vi "zad_14.vi"() -> ()   [LabVIEW 2024]
uses:
  Data_14.ctl
  <vilib>/regexp/Match Regular Expression.xnode
panel:
  out "error out":errorcluster
  in  "error in":errorcluster
  out "Limit exceeded?":bool
  out "To be moved":string
  in  "Sound intensity: MAX":dbl=100.0
  in  "Sound intensity: MIN":dbl
  in  "Stop":bool
  in  "Sound intensity [dB]":dbl(slide) scale=0.0..100.0
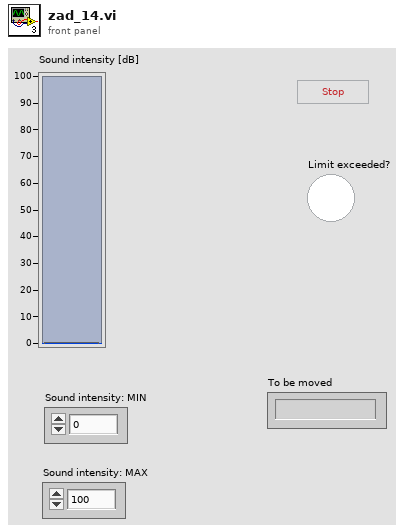
[diagram p1: front panel]
types:
  T1 = typedef "Data_14.ctl" = cluster{"Left":i32, "Top":i32, "Dragging":bool, "Letters":string}
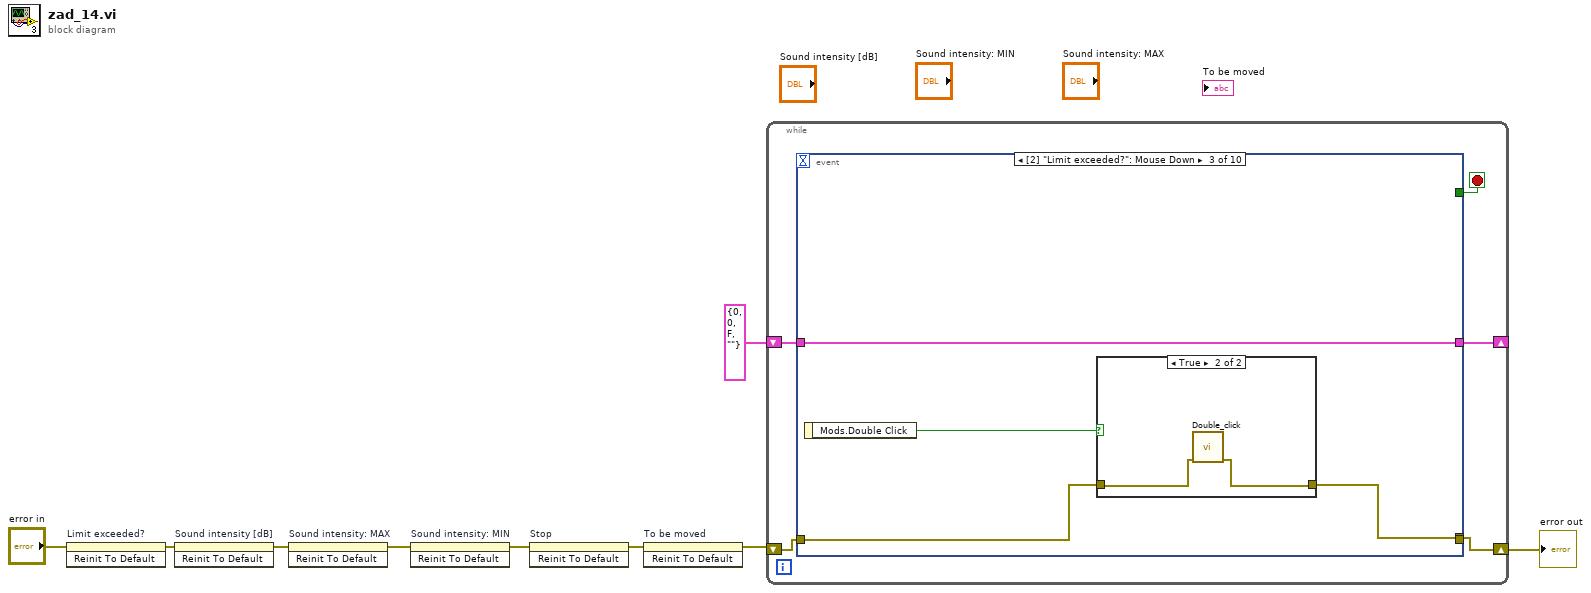
[diagram p0: block diagram]
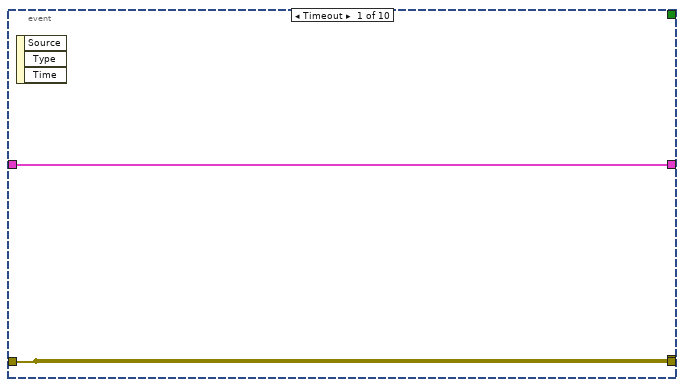
[diagram p2: hidden frame]
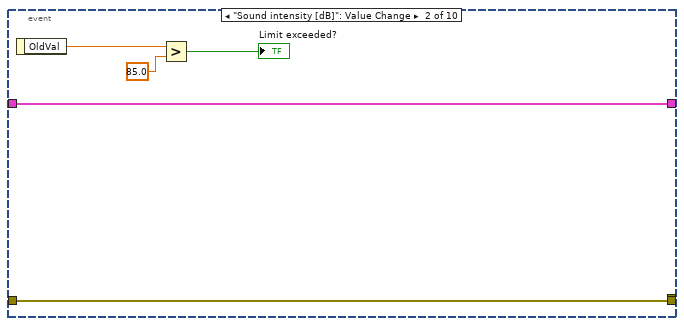
[diagram p3: hidden frame]
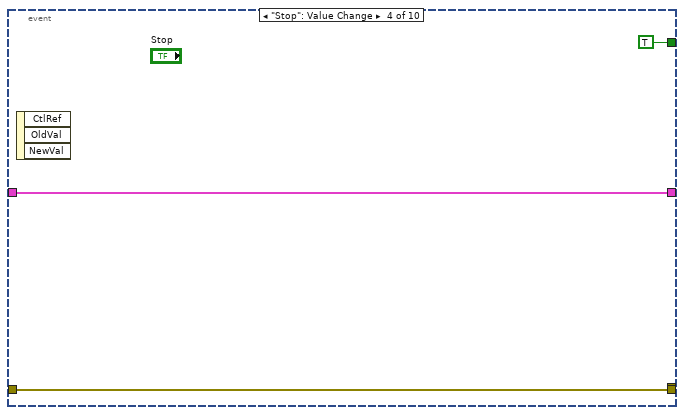
[diagram p5: hidden frame]
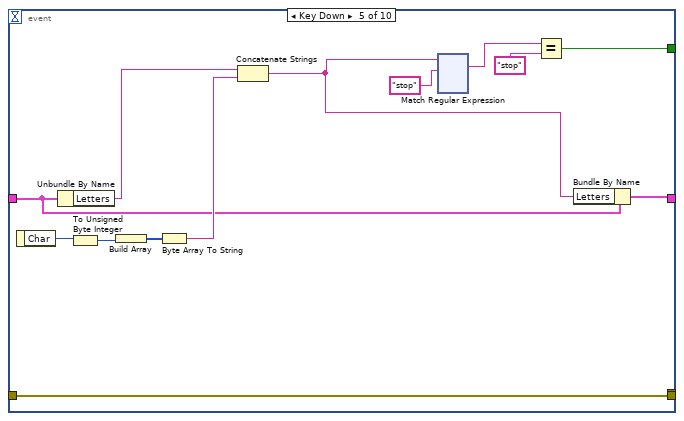
[diagram p6: hidden frame]
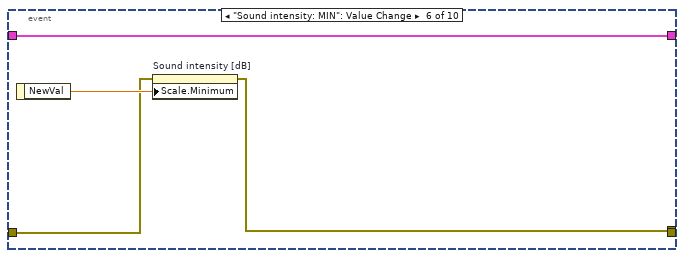
[diagram p7: hidden frame]
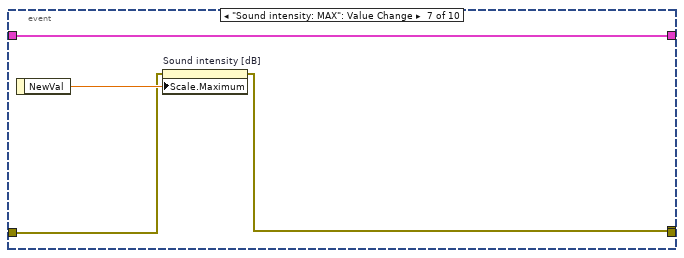
[diagram p8: hidden frame]
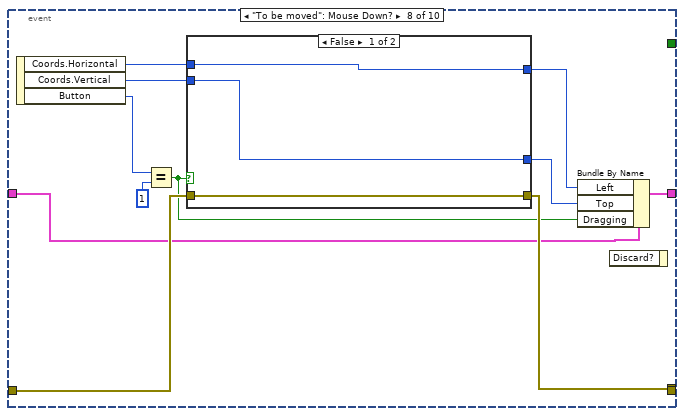
[diagram p9: hidden frame]
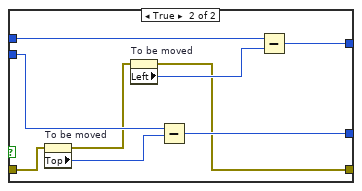
[diagram p10: hidden frame]
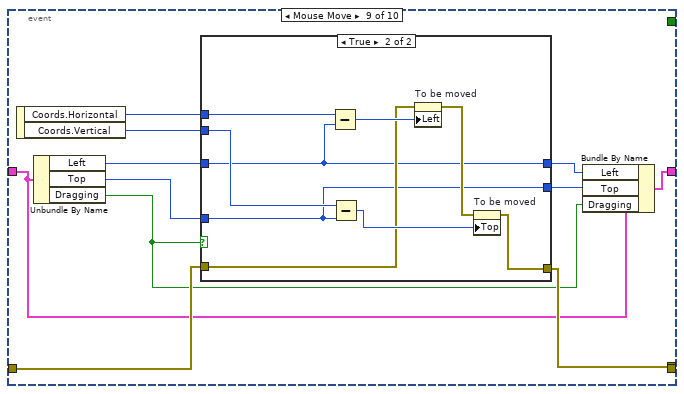
[diagram p11: hidden frame]
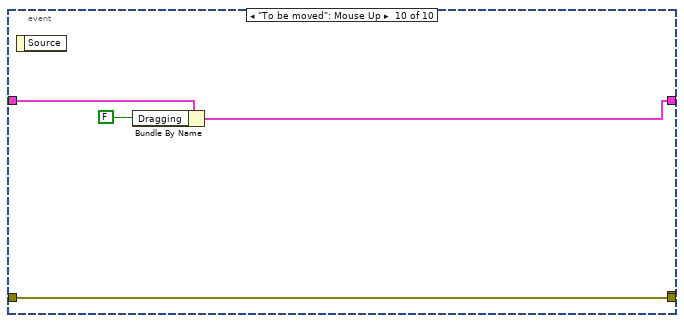
[diagram p13: hidden frame]
diagram:
  n1 = invoke on="Limit exceeded?" class="Bool (strict)" method="Reinit To Default"(error in="error in") -> (error out=w5:errorcluster)  [unwired: 2 in, 2 out]
  n2 = invoke on="Sound intensity [dB]" class="Slide (strict)" method="Reinit To Default"(error in=w5) -> (error out=w6:errorcluster)  [unwired: 2 in, 2 out]
  n3 = invoke on="Sound intensity: MAX" class="DigNum (strict)" method="Reinit To Default"(error in=w6) -> (error out=w7:errorcluster)  [unwired: 2 in, 2 out]
  n4 = invoke on="Sound intensity: MIN" class="DigNum (strict)" method="Reinit To Default"(error in=w7) -> (error out=w8:errorcluster)  [unwired: 2 in, 2 out]
  n5 = invoke on="Stop" class="Bool" method="Reinit To Default"(error in=w8) -> (error out=w9:errorcluster)  [unwired: 2 in, 2 out]
  n6 = invoke on="To be moved" class="Str" method="Reinit To Default"(error in=w9) -> (error out=w2:errorcluster)  [unwired: 2 in, 2 out]
  n7 = while {
    shift-right: [w12] -> w3
    shift-left: w2 -> [w13]
    shift-right: [w10] -> _
    shift-left: T1 {"Left"=0, "Top"=0, "Dragging"=FALSE, "Letters"=""} -> [w11]
    stop <- w14 stop-if-true
    n8 = event shown="[2] \"Limit exceeded?\": Mouse Down" {
      selector: _ -> [_ _ _ _ _ _ _ _ _ _]
      dyn-events: _ -> [_ _ _ _ _ _ _ _ _ _]
      timeout: _ -> [_ _ _ _ _ _ _ _ _ _]
      tunnel: [_ _ _ TRUE w40 _ _ _ _ _] -> w14
      tunnel: w13 -> [w16 w18 w25 w30 w44 w164 w168 w176 w203 w219]
      tunnel: [w16 w18 w24 w30 w44 w163 w167 w175 w202 w219] -> w12
      tunnel: [w16 _ _ _ _ _ _ _ _ _] -> _
      tunnel: w11 -> [w15 w17 w22 w29 w34 w162 w166 w174 w197 w218]
      tunnel: [w15 w17 w22 w29 w32 w162 w166 w171 w194 w216] -> w10
      event Timeout {
        n9 = event-data() -> ()  [unwired: 1 in, 3 out]
      }
      event "Sound intensity [dB]": Value Change {
        n10 = event-data() -> ("OldVal"=w21:dbl)  [unwired: 1 in]
        n11 = Greater?(x=w21, y=85.0) -> (0:→"Limit exceeded?":bool)
      }
      event "Limit exceeded?": Mouse Down {
        n12 = event-data() -> ("Mods.Double Click"=w23:bool)  [unwired: 1 in]
        n13 = case shown="True" w23 {
          tunnel: w25 -> [w26 w28]
          tunnel: [w26 w27] -> w24
          frame False {
          }
          frame True {
            n14 = call "Double_click.vi"("error in"=w28) -> ("error out"=w27:errorcluster)  [unwired: 10 in]
          }
        }
      }
      event "Stop": Value Change {
        n15 = event-data() -> ()  [unwired: 1 in, 3 out]
      }
      event Key Down {
        n16 = event-data() -> ("Char"=w39:i16)  [unwired: 1 in]
        n17 = Unbundle By Name(w34) -> ("Letters"=w35:string)
        n18 = To Unsigned Byte Integer(number=w39) -> (unsigned 8bit integer=w38:u8)
        n19 = Build Array(w38) -> (w37:u8[])
        n20 = Byte Array To String(unsigned byte array=w37) -> (string=w36:string)
        n21 = Concatenate Strings(w35, w36) -> (w33:string)
        n22 = xnode "Match Regular Expression"("input string"=w33, "regular expression"="stop") -> ("whole match"=w42:string)  [unwired: 4 in, 4 out]
        n23 = Equal?(x=w42, y="stop") -> (x = y?=w40:bool)
        n24 = Bundle By Name(cluster=w34, "Letters"=w33) -> (w32:T1)
      }
      event "Sound intensity: MIN": Value Change {
        n25 = event-data() -> ("NewVal"=w165:dbl)  [unwired: 1 in]
        n26 = property on="Sound intensity [dB]" class="Slide (strict)"(error in=w164, "Scale.Minimum"=w165) -> (error out=w163:errorcluster)  [unwired: 1 in, 1 out]
      }
      event "Sound intensity: MAX": Value Change {
        n27 = event-data() -> ("NewVal"=w169:dbl)  [unwired: 1 in]
        n28 = property on="Sound intensity [dB]" class="Slide (strict)"(error in=w168, "Scale.Maximum"=w169) -> (error out=w167:errorcluster)  [unwired: 1 in, 1 out]
      }
      event "To be moved": Mouse Down? {
        n29 = event-data() -> ("Coords.Horizontal"=w180:i32, "Coords.Vertical"=w179:i32, "Button"=w178:u16)  [unwired: 1 in]
        n30 = Equal?(x=w178, y=u16 1) -> (x = y?=w170:bool)
        n31 = case shown="False" w170 {
          tunnel: w180 -> [w182 w192]
          tunnel: w179 -> [w183 w191]
          tunnel: [w183 w190] -> w173
          tunnel: [w182 w189] -> w172
          tunnel: w176 -> [w181 w186]
          tunnel: [w181 w184] -> w175
          frame False {
          }
          frame True {
            n32 = property on="To be moved" class="Str"(error in=w186) -> (error out=w185:errorcluster, "Top"=w187:i32)  [unwired: 1 in, 1 out]
            n33 = property on="To be moved" class="Str"(error in=w185) -> (error out=w184:errorcluster, "Left"=w188:i32)  [unwired: 1 in, 1 out]
            n34 = Subtract(x=w191, y=w187) -> (x-y=w190:i32)
            n35 = Subtract(x=w192, y=w188) -> (x-y=w189:i32)
          }
        }
        n36 = Bundle By Name(cluster=w174, "Left"=w172, "Top"=w173, "Dragging"=w170) -> (w171:T1)
        n37 = event-data() -> ()  [unwired: 2 in, 1 out]
      }
      event Mouse Move {
        n38 = event-data() -> ("Coords.Horizontal"=w201:i32, "Coords.Vertical"=w200:i32)  [unwired: 1 in]
        n39 = Unbundle By Name(w197) -> ("Left"=w199:i32, "Top"=w198:i32, "Dragging"=w193:bool)
        n40 = case shown="True" w193 {
          tunnel: w203 -> [w206 w210]
          tunnel: [w206 w215] -> w202
          tunnel: w201 -> [_ w214]
          tunnel: w200 -> [_ w213]
          tunnel: w199 -> [w205 w208]
          tunnel: w198 -> [w204 w207]
          tunnel: [w205 w208] -> w196
          tunnel: [w204 w207] -> w195
          frame False {
          }
          frame True {
            n41 = Subtract(x=w214, y=w208) -> (x-y=w212:i32)
            n42 = Subtract(x=w213, y=w207) -> (x-y=w211:i32)
            n43 = property on="To be moved" class="Str"(error in=w210, "Left"=w212) -> (error out=w209:errorcluster)  [unwired: 1 in, 1 out]
            n44 = property on="To be moved" class="Str"(error in=w209, "Top"=w211) -> (error out=w215:errorcluster)  [unwired: 1 in, 1 out]
          }
        }
        n45 = Bundle By Name(cluster=w197, "Left"=w196, "Top"=w195, "Dragging"=w193) -> (w194:T1)
      }
      event "To be moved": Mouse Up {
        n46 = event-data() -> ()  [unwired: 1 in, 1 out]
        n47 = Bundle By Name(cluster=w218, "Dragging"=FALSE) -> (w216:T1)
      }
    }
  }
  "error out" <- w3
